vi "Call ADB.vi"(3 "error in":errorcluster, 4 "adb sub-command":string, 5 "adb location":string) -> (0 "error out":errorcluster, 1 "standard error":string, 2 "standard output":string)   [LabVIEW 2016]
doc: "Calls the ADB command line utility at \"adb location\" or default /usr/bin/adb with \"adb sub-command\". The \"adb sub-command\" should include all arguements formatted as appropriate for a command line utility."
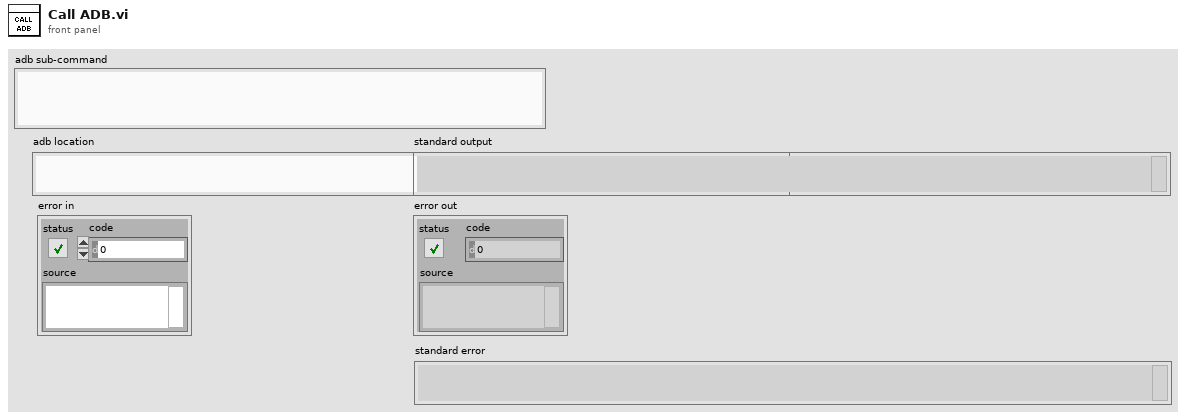
[diagram p1: front panel]
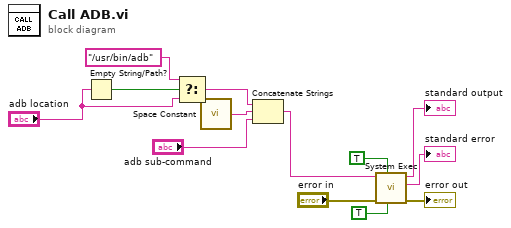
[diagram p0: block diagram]
diagram:
  n1 = Empty String/Path?(string/path="adb location") -> (empty?=w12:bool)
  n2 = Select(t="/usr/bin/adb" ("name or relative path"), s=w12, f="adb location") -> (s? t:f=w3:string)
  n3 = call <vilib>:"Space Constant.vi"() -> ("String"=w5:string)
  n4 = Concatenate Strings(w3, w5, "adb sub-command") -> (w2:string)
  n5 = call <vilib>:"System Exec.vi"("run minimized? (F)"=TRUE, "wait until completion? (T)"=TRUE, "error in (no error)"="error in", "command line"=w2) -> ("error out"=→"error out":errorcluster, "standard error"=→"standard error":string, "standard output"=→"standard output":string)  [unwired: 4 in, 1 out]
